vi "Write Minimum speed.vi"(8 "error in (no error)":errorcluster, 10 "Minimum speed":dbl, 11 "Motor-Analog in":refnum<class "Motor-Analog.lvclass">) -> (0 "error out":errorcluster, 3 "Motor-Analog out":refnum<class "Motor-Analog.lvclass">)   [LabVIEW 2013, in "PowderDeposition.lvlib" / "Motor-Analog.lvclass"]
uses:
  Motor-Analog.lvclass
  Motor-Analog.lvclass/Motor-Analog.ctl
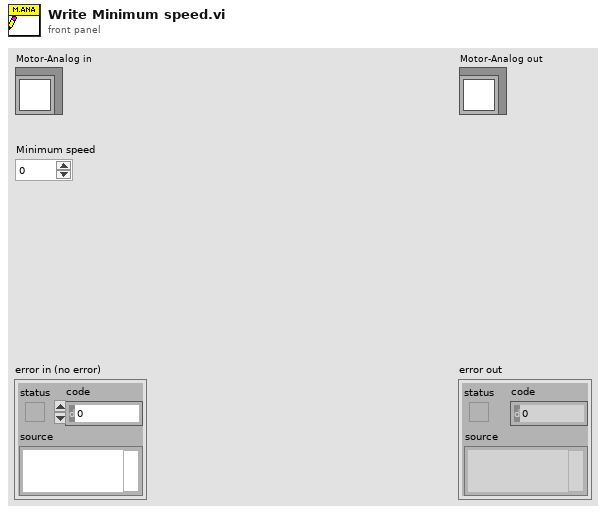
[diagram p1: front panel]
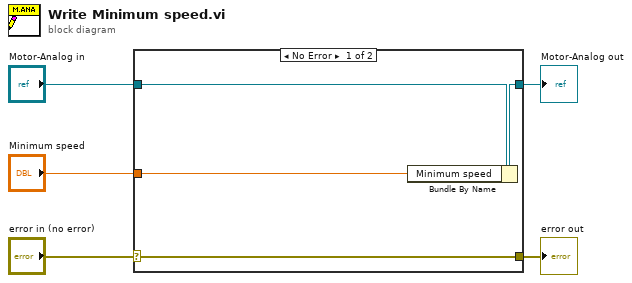
[diagram p0: block diagram]
diagram:
  n1 = case shown="No Error" "error in (no error)" {
    selector: "error in (no error)" -> [w9 w10]
    tunnel: [w9 w10] -> w4
    tunnel: [w7 w11] -> w2
    tunnel: "Motor-Analog in" -> [w8 w11]
    tunnel: "Minimum speed" -> [w6 _]
    frame No Error {
      n2 = Bundle By Name(cluster=w8, "Minimum speed"=w6) -> (w7:refnum<class "Motor-Analog.lvclass">)
    }
    frame Error {
    }
  }
  "error out" <- w4
  "Motor-Analog out" <- w2
